vi "create.vi"(8 "error in":errorcluster) -> (0 "error out":errorcluster, 3 "event reporter out":refnum<class "event reporter.lvclass">)   [LabVIEW 2013, in "event reporter.lvclass"]
uses:
  event reporter.lvclass
  result/result.lvclass
  event reporter.lvclass/event reporter.ctl
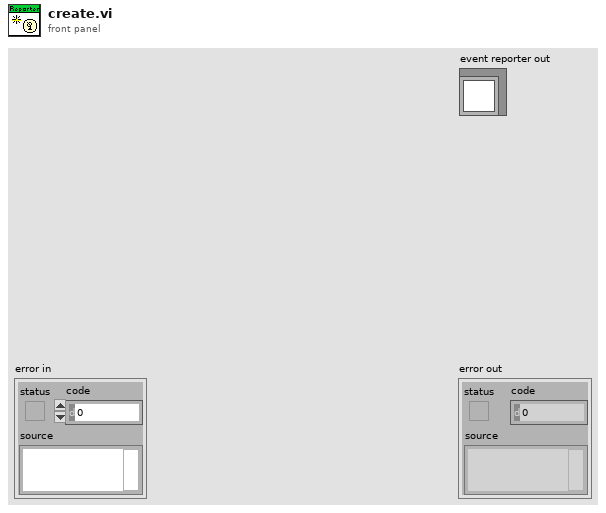
[diagram p1: front panel]
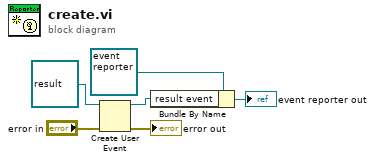
[diagram p0: block diagram]
diagram:
  n1 = Create User Event(user event datatype=refnum<class "result.lvclass"> refnum ("result"), error in="error in") -> (user event=w1:refnum<user-event>, error out=→"error out":errorcluster)
  n2 = Bundle By Name(cluster=refnum<class "event reporter.lvclass"> refnum ("event reporter in"), "result event"=w1) -> (→"event reporter out":refnum<class "event reporter.lvclass">)
